vi "JSON File Parse String.vi"(8 "error in (no error)":errorcluster, 11 "file json string":string) -> (0 "error out":errorcluster, 1 "version substring":string, 2 "dsf version substring":string, 3 "dsf configuration substring":string)   [LabVIEW 2020, in "DSF Core.lvlib" / "Configuration Session.lvclass"]
uses:
  Configuration Session.lvclass
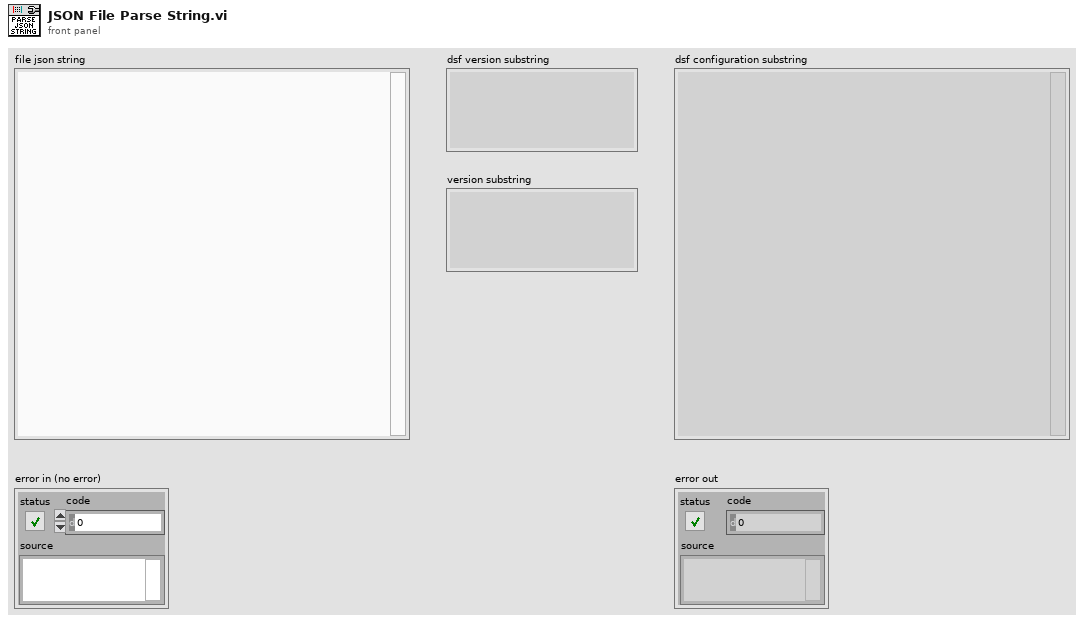
[diagram p1: front panel]
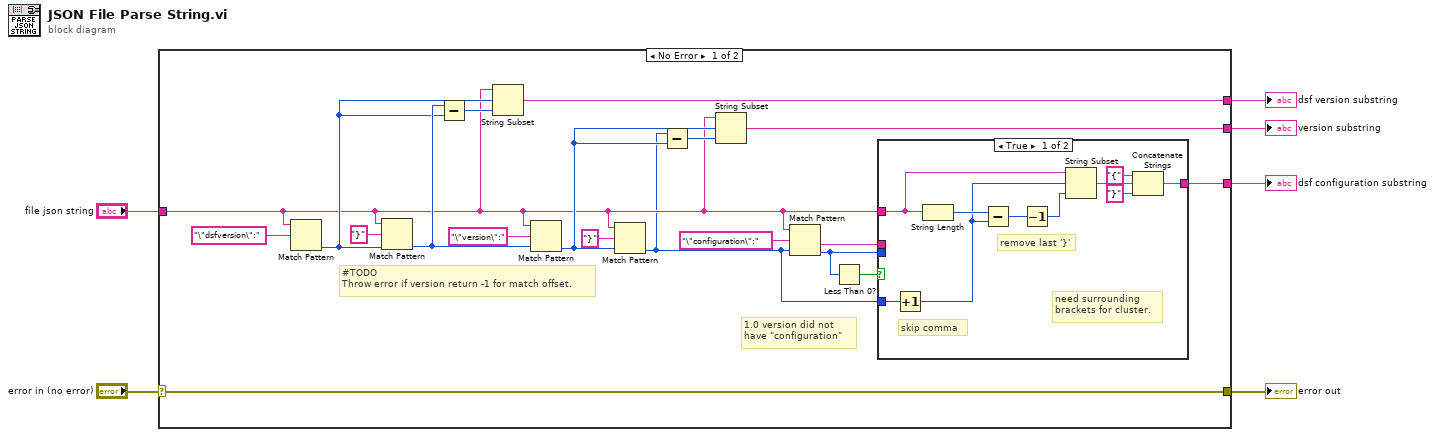
[diagram p0: block diagram]
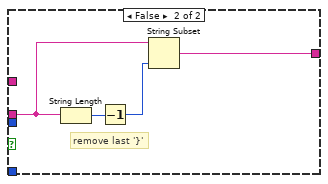
[diagram p2: hidden frame]
diagram:
  n1 = case shown="No Error" "error in (no error)" {
    selector: "error in (no error)" -> [w15 w40]
    tunnel: [w9 _] -> w6
    tunnel: "file json string" -> [w10 _]
    tunnel: [w18 _] -> w4
    tunnel: [w17 _] -> w3
    tunnel: [w15 w40] -> w1
    frame No Error {
      # "1.0 version did not have \"configuration\""
      # "#TODO\nThrow error if version return -1 for match offset."
      n2 = Match Pattern(string=w10, regular expression="\"dsfversion\":") -> (offset past match=w20:i32)  [unwired: 1 in, 3 out]
      n3 = Match Pattern(string=w10, regular expression="}", offset (0)=w20) -> (offset past match=w21:i32)  [unwired: 3 out]
      n4 = Subtract(x=w21, y=w20) -> (x-y=w19:i32)
      n5 = String Subset(string=w10, offset (0)=w20, length (rest)=w19) -> (substring=w18:string)
      n6 = Match Pattern(string=w10, regular expression="\"version\":", offset (0)=w21) -> (offset past match=w14:i32)  [unwired: 3 out]
      n7 = Match Pattern(string=w10, regular expression="}", offset (0)=w14) -> (offset past match=w7:i32)  [unwired: 3 out]
      n8 = Subtract(x=w7, y=w14) -> (x-y=w22:i32)
      n9 = String Subset(string=w10, offset (0)=w14, length (rest)=w22) -> (substring=w17:string)
      n10 = Match Pattern(string=w10, regular expression="\"configuration\":", offset (0)=w7) -> (after substring=w8:string, offset past match=w11:i32)  [unwired: 2 out]
      n11 = Less Than 0?(x=w11) -> (x < 0?=w12:bool)
      n12 = case shown="True" w12 {
        tunnel: w11 -> [_ _]
        tunnel: w10 -> [w33 _]
        tunnel: [w26 w38] -> w9
        tunnel: w8 -> [_ w37]
        tunnel: w7 -> [w34 _]
        frame True {
          # "need surrounding brackets for cluster."
          # "skip comma"
          # "remove last '}'"
          n13 = Increment(x=w34) -> (x+1=w31:i32)
          n14 = String Length(string=w33) -> (length=w32:i32)
          n15 = Subtract(x=w32, y=w31) -> (x-y=w30:i32)
          n16 = Decrement(x=w30) -> (x-1=w35:i32)
          n17 = String Subset(string=w33, offset (0)=w31, length (rest)=w35) -> (substring=w27:string)
          n18 = Concatenate Strings("{" ("string"), w27, "}" ("string")) -> (w26:string)
        }
        frame False {
          # "remove last '}'"
          n19 = String Length(string=w37) -> (length=w39:i32)
          n20 = Decrement(x=w39) -> (x-1=w36:i32)
          n21 = String Subset(string=w37, length (rest)=w36) -> (substring=w38:string)  [unwired: 1 in]
        }
      }
    }
    frame Error {
    }
  }
  "dsf version substring" <- w4
  "dsf configuration substring" <- w6
  "version substring" <- w3
  "error out" <- w1
